vi "sub_GetNextState.vi"(4 "Stop":bool, 5 "Elapsed Time (sec)":dbl format="%#.2g", 6 "Start":bool, 7 "Car Position Slider":T1 scale=0.0..4.0, 8 "error in":errorcluster caption="에러 입력", 10 "Wash Options":T2, 11 "CurrentState":T3) -> (0 "error out":errorcluster caption="에러 출력", 3 "NextState":T3)   [LabVIEW 2018]
uses:
  Control/WashState.ctl
  Control/Wash Options.ctl
  Control/Car Position Control.ctl
  Control/Time.ctl
panel:
  out "결과":bool
  # "0"
  # "1"
  # "2"
  # "3"
  # "4"
  # "5"
  # "6"
  # "7"
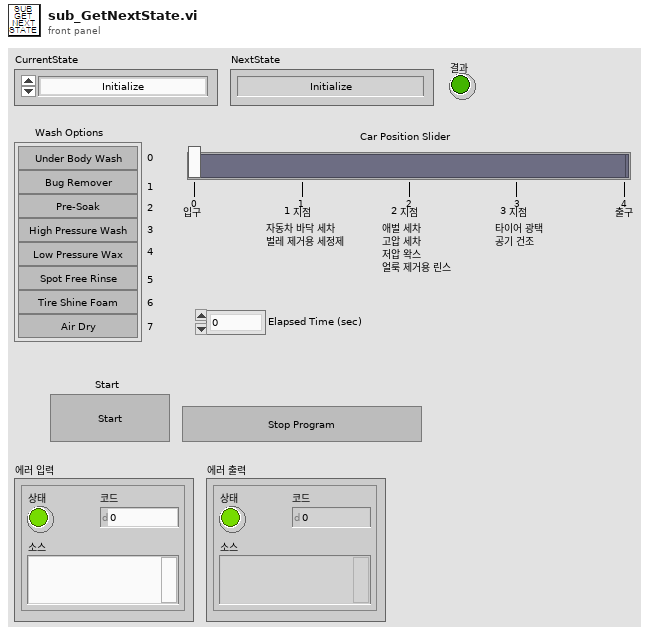
[diagram p1: front panel]
types:
  T1 = typedef "Car Position Control.ctl" = i32
  T2 = typedef "Wash Options.ctl" = cluster{"Under Body Wash":bool, "Bug Remover":bool, "Pre-Soak":bool, "High Pressure Wash":bool, "Low Pressure Wax":bool, "Spot Free Rinse":bool, "Tire Shine Foam":bool, "Air Dry":bool}
  T3 = typedef "WashState.ctl" = enum16{"Initialize", "Ready", "Under Body Wash", "Bug Remover", "Pre-Soak", "High Pressure Wash", "Low Pressure Wax", "Spot Free Rinse", "Tire Shine Foam", "Air Dry", "Stop", "Exit"}
  T4 = typedef "Time.ctl" = enum16{"Start", "End"}
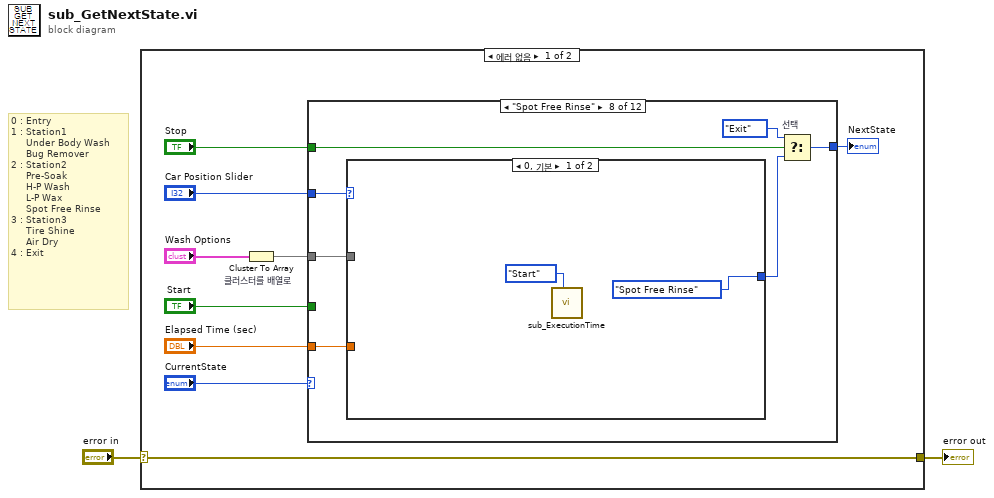
[diagram p0: block diagram]
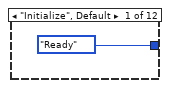
[diagram p2: hidden frame]
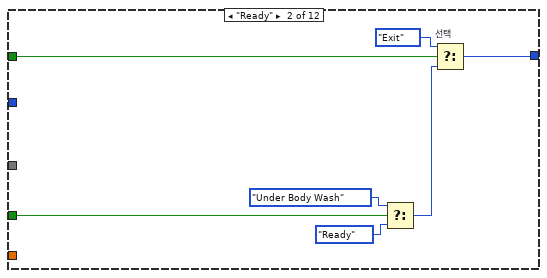
[diagram p3: hidden frame]
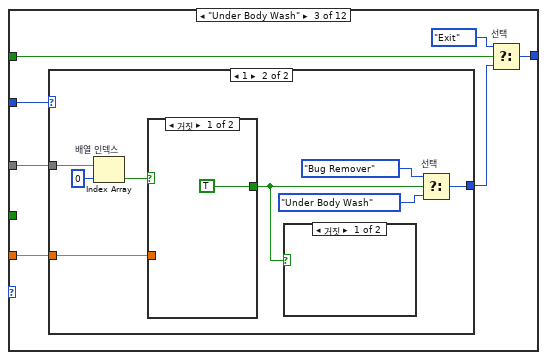
[diagram p4: hidden frame]
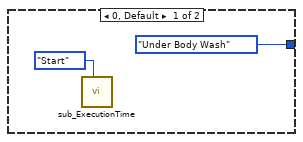
[diagram p5: hidden frame]
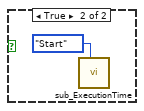
[diagram p6: hidden frame]
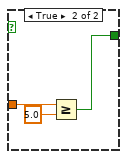
[diagram p7: hidden frame]
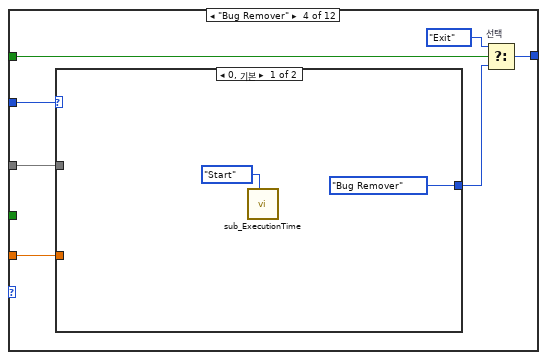
[diagram p8: hidden frame]
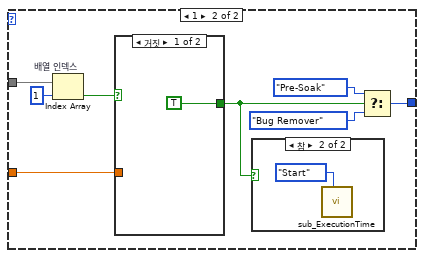
[diagram p9: hidden frame]
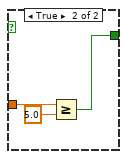
[diagram p11: hidden frame]
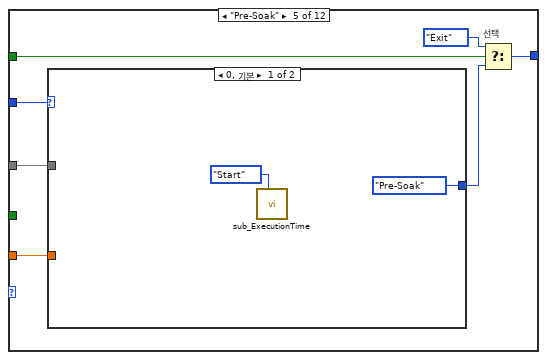
[diagram p12: hidden frame]
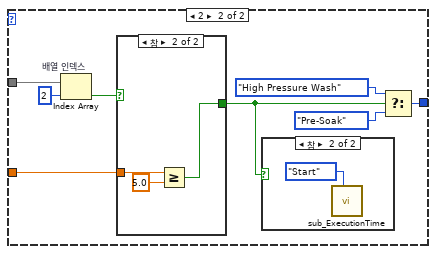
[diagram p13: hidden frame]
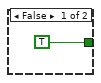
[diagram p15: hidden frame]
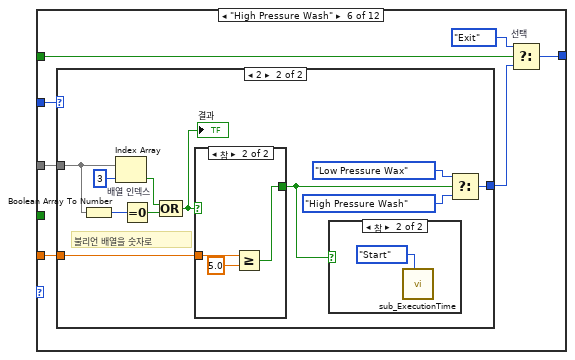
[diagram p16: hidden frame]
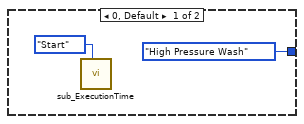
[diagram p17: hidden frame]
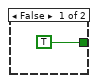
[diagram p19: hidden frame]
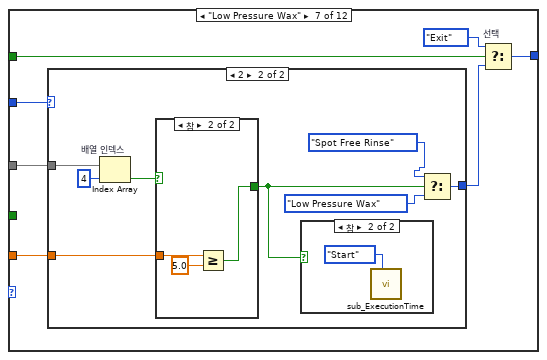
[diagram p20: hidden frame]
diagram:
  # "0 : Entry\n1 : Station1\n     Under Body Wash\n     Bug Remover\n2 : Station2\n     Pre-Soak\n     H-P Wash\n     L-P Wax\n     Spot Free Rinse\n3 : Station3\n     Tire Shine\n     Air Dry\n4 : Exit"
  n1 = case shown="에러 없음" "error in" {
    selector: "error in" -> [w11 w207]
    tunnel: [w11 w207] -> w1
    frame No Error {
      n2 = Cluster To Array "클러스터를 배열로"(cluster="Wash Options") -> (array=w7:bool[])
      n3 = case shown="\"Spot Free Rinse\"" "CurrentState" {
        tunnel: [WashState."Ready" ("NextState") w18 w25 w47 w69 w91 w116 w138 w160 w182 w202 WashState."Exit" ("NextState")] -> w9
        tunnel: w7 -> [_ _ w23 w45 w67 w89 w114 w136 w158 w180 _ _]
        tunnel: "Start" -> [_ w13 _ _ _ _ _ _ _ _ _ _]
        tunnel: "Stop" -> [_ w19 w26 w48 w70 w92 w117 w139 w161 w183 w203 _]
        tunnel: "Car Position Slider" -> [_ _ w21 w43 w65 w87 w112 w134 w156 w178 w199 _]
        tunnel: "Elapsed Time (sec)" -> [_ _ w20 w42 w64 w86 w111 w133 w155 w177 _ _]
        frame "Initialize", Default {
        }
        frame "Ready" {
          n4 = Select(t=WashState."Under Body Wash" ("NextState"), s=w13, f=WashState."Ready" ("NextState")) -> (s? t:f=w15:T3)
          n5 = Select "선택"(t=WashState."Exit" ("NextState"), s=w19, f=w15) -> (s? t:f=w18:T3)
        }
        frame "Under Body Wash" {
          n6 = case shown="1" w21 {
            tunnel: w23 -> [_ w36]
            tunnel: [WashState."Under Body Wash" ("NextState") w31] -> w22
            tunnel: w20 -> [_ w30]
            frame 0, Default {
              n7 = call "sub_ExecutionTime.vi"("State"=Time."Start") -> ()  [unwired: 9 in, 2 out]
            }
            frame 1 {
              n8 = Index Array "배열 인덱스"(array=w36, index=0 ("인덱스")) -> (element=w34:bool)
              n9 = case shown="거짓" w34 {
                tunnel: [TRUE ("Finish?") w39] -> w29
                tunnel: w30 -> [_ w41]
                frame False {
                }
                frame True {
                  n10 = Greater Or Equal?(x=w41, y=5.0) -> (x >= y?=w39:bool)
                }
              }
              n11 = case shown="거짓" w29 {
                frame False {
                }
                frame True {
                  n12 = call "sub_ExecutionTime.vi"("State"=Time."Start") -> ()  [unwired: 9 in, 2 out]
                }
              }
              n13 = Select "선택"(t=WashState."Bug Remover" ("NextState"), s=w29, f=WashState."Under Body Wash" ("NextState")) -> (s? t:f=w31:T3)
            }
          }
          n14 = Select "선택"(t=WashState."Exit" ("NextState"), s=w26, f=w22) -> (s? t:f=w25:T3)
        }
        frame "Bug Remover" {
          n15 = case shown="0, 기본" w43 {
            tunnel: w45 -> [_ w58]
            tunnel: [WashState."Bug Remover" ("NextState") w52] -> w44
            tunnel: w42 -> [_ w56]
            frame 0, Default {
              n16 = call "sub_ExecutionTime.vi"("State"=Time."Start") -> ()  [unwired: 9 in, 2 out]
            }
            frame 1 {
              n17 = Index Array "배열 인덱스"(array=w58, index=1 ("인덱스")) -> (element=w55:bool)
              n18 = case shown="거짓" w55 {
                tunnel: [TRUE ("Finish?") w61] -> w51
                tunnel: w56 -> [_ w63]
                frame False {
                }
                frame True {
                  n19 = Greater Or Equal?(x=w63, y=5.0) -> (x >= y?=w61:bool)
                }
              }
              n20 = case shown="참" w51 {
                frame False {
                }
                frame True {
                  n21 = call "sub_ExecutionTime.vi"("State"=Time."Start") -> ()  [unwired: 9 in, 2 out]
                }
              }
              n22 = Select(t=WashState."Pre-Soak" ("NextState"), s=w51, f=WashState."Bug Remover" ("NextState")) -> (s? t:f=w52:T3)
            }
          }
          n23 = Select "선택"(t=WashState."Exit" ("NextState"), s=w48, f=w44) -> (s? t:f=w47:T3)
        }
        frame "Pre-Soak" {
          n24 = case shown="0, 기본" w65 {
            tunnel: w67 -> [_ w80]
            tunnel: [WashState."Pre-Soak" ("NextState") w74] -> w66
            tunnel: w64 -> [_ w77]
            frame 0, Default {
              n25 = call "sub_ExecutionTime.vi"("State"=Time."Start") -> ()  [unwired: 9 in, 2 out]
            }
            frame 2 {
              n26 = Index Array "배열 인덱스"(array=w80, index=2 ("인덱스")) -> (element=w78:bool)
              n27 = case shown="참" w78 {
                tunnel: [TRUE ("Finish?") w83] -> w73
                tunnel: w77 -> [_ w85]
                frame False {
                }
                frame True {
                  n28 = Greater Or Equal?(x=w85, y=5.0) -> (x >= y?=w83:bool)
                }
              }
              n29 = case shown="참" w73 {
                frame False {
                }
                frame True {
                  n30 = call "sub_ExecutionTime.vi"("State"=Time."Start") -> ()  [unwired: 9 in, 2 out]
                }
              }
              n31 = Select(t=WashState."High Pressure Wash" ("NextState"), s=w73, f=WashState."Pre-Soak" ("NextState")) -> (s? t:f=w74:T3)
            }
          }
          n32 = Select "선택"(t=WashState."Exit" ("NextState"), s=w70, f=w66) -> (s? t:f=w69:T3)
        }
        frame "High Pressure Wash" {
          n33 = case shown="2" w87 {
            tunnel: w89 -> [_ w99]
            tunnel: [WashState."High Pressure Wash" ("NextState") w101] -> w88
            tunnel: w86 -> [_ w104]
            frame 0, Default {
              n34 = call "sub_ExecutionTime.vi"("State"=Time."Start") -> ()  [unwired: 9 in, 2 out]
            }
            frame 2 {
              # "불리언 배열을 숫자로"
              n35 = Boolean Array To Number(Boolean array=w99) -> (number=w98:u32)
              n36 = Index Array "배열 인덱스"(array=w99, index=3 ("인덱스")) -> (element=w97:bool)
              n37 = Equal To 0?(x=w98) -> (x = 0?=w96:bool)
              n38 = Compound Arithmetic op=OR(w97, w96) -> (w95:bool)
              "결과" <- w95
              n39 = case shown="참" w95 {
                tunnel: [TRUE ("Finish?") w108] -> w100
                tunnel: w104 -> [_ w110]
                frame False {
                }
                frame True {
                  n40 = Greater Or Equal?(x=w110, y=5.0) -> (x >= y?=w108:bool)
                }
              }
              n41 = case shown="참" w100 {
                frame False {
                }
                frame True {
                  n42 = call "sub_ExecutionTime.vi"("State"=Time."Start") -> ()  [unwired: 9 in, 2 out]
                }
              }
              n43 = Select(t=WashState."Low Pressure Wax" ("NextState"), s=w100, f=WashState."High Pressure Wash" ("NextState")) -> (s? t:f=w101:T3)
            }
          }
          n44 = Select "선택"(t=WashState."Exit" ("NextState"), s=w92, f=w88) -> (s? t:f=w91:T3)
        }
        frame "Low Pressure Wax" {
          n45 = case shown="2" w112 {
            tunnel: w114 -> [_ w127]
            tunnel: [WashState."Low Pressure Wax" ("NextState") w122] -> w113
            tunnel: w111 -> [_ w124]
            frame 0, Default {
              n46 = call "sub_ExecutionTime.vi"("State"=Time."Start") -> ()  [unwired: 9 in, 2 out]
            }
            frame 2 {
              n47 = Index Array "배열 인덱스"(array=w127, index=4 ("인덱스")) -> (element=w125:bool)
              n48 = case shown="참" w125 {
                tunnel: [TRUE ("Finish?") w130] -> w121
                tunnel: w124 -> [_ w132]
                frame False {
                }
                frame True {
                  n49 = Greater Or Equal?(x=w132, y=5.0) -> (x >= y?=w130:bool)
                }
              }
              n50 = case shown="참" w121 {
                frame False {
                }
                frame True {
                  n51 = call "sub_ExecutionTime.vi"("State"=Time."Start") -> ()  [unwired: 9 in, 2 out]
                }
              }
              n52 = Select(t=WashState."Spot Free Rinse" ("NextState"), s=w121, f=WashState."Low Pressure Wax" ("NextState")) -> (s? t:f=w122:T3)
            }
          }
          n53 = Select "선택"(t=WashState."Exit" ("NextState"), s=w117, f=w113) -> (s? t:f=w116:T3)
        }
        frame "Spot Free Rinse" {
          n54 = case shown="0, 기본" w134 {
            tunnel: w136 -> [_ w149]
            tunnel: [WashState."Spot Free Rinse" ("NextState") w144] -> w135
            tunnel: w133 -> [_ w146]
            frame 0, Default {
              n55 = call "sub_ExecutionTime.vi"("State"=Time."Start") -> ()  [unwired: 9 in, 2 out]
            }
            frame 2 {
              n56 = Index Array "배열 인덱스"(array=w149, index=5 ("인덱스")) -> (element=w147:bool)
              n57 = case shown="참" w147 {
                tunnel: [TRUE ("Finish?") w152] -> w143
                tunnel: w146 -> [_ w154]
                frame False {
                }
                frame True {
                  n58 = Greater Or Equal?(x=w154, y=5.0) -> (x >= y?=w152:bool)
                }
              }
              n59 = case shown="참" w143 {
                frame False {
                }
                frame True {
                  n60 = call "sub_ExecutionTime.vi"("State"=Time."Start") -> ()  [unwired: 9 in, 2 out]
                }
              }
              n61 = Select(t=WashState."Tire Shine Foam" ("NextState"), s=w143, f=WashState."Spot Free Rinse" ("NextState")) -> (s? t:f=w144:T3)
            }
          }
          n62 = Select "선택"(t=WashState."Exit" ("NextState"), s=w139, f=w135) -> (s? t:f=w138:T3)
        }
        frame "Tire Shine Foam" {
          n63 = case shown="0, 기본" w156 {
            tunnel: w158 -> [_ w171]
            tunnel: [WashState."Tire Shine Foam" ("NextState") w165] -> w157
            tunnel: w155 -> [_ w168]
            frame 0, Default {
              n64 = call "sub_ExecutionTime.vi"("State"=Time."Start") -> ()  [unwired: 9 in, 2 out]
            }
            frame 3 {
              n65 = Index Array "배열 인덱스"(array=w171, index=6 ("인덱스")) -> (element=w169:bool)
              n66 = case shown="참" w169 {
                tunnel: [TRUE ("Finish?") w174] -> w164
                tunnel: w168 -> [_ w176]
                frame False {
                }
                frame True {
                  n67 = Greater Or Equal?(x=w176, y=5.0) -> (x >= y?=w174:bool)
                }
              }
              n68 = case shown="참" w164 {
                frame False {
                }
                frame True {
                  n69 = call "sub_ExecutionTime.vi"("State"=Time."Start") -> ()  [unwired: 9 in, 2 out]
                }
              }
              n70 = Select(t=WashState."Air Dry" ("NextState"), s=w164, f=WashState."Tire Shine Foam" ("NextState")) -> (s? t:f=w165:T3)
            }
          }
          n71 = Select "선택"(t=WashState."Exit" ("NextState"), s=w161, f=w157) -> (s? t:f=w160:T3)
        }
        frame "Air Dry" {
          n72 = case shown="0, 기본" w178 {
            tunnel: w180 -> [_ w193]
            tunnel: [WashState."Air Dry" ("NextState") w187] -> w179
            tunnel: w177 -> [_ w190]
            frame 0, Default {
              n73 = call "sub_ExecutionTime.vi"("State"=Time."Start") -> ()  [unwired: 9 in, 2 out]
            }
            frame 3 {
              n74 = Index Array "배열 인덱스"(array=w193, index=7 ("인덱스")) -> (element=w191:bool)
              n75 = case shown="참" w191 {
                tunnel: [TRUE ("Finish?") w196] -> w186
                tunnel: w190 -> [_ w198]
                frame False {
                }
                frame True {
                  n76 = Greater Or Equal?(x=w198, y=5.0) -> (x >= y?=w196:bool)
                }
              }
              n77 = case shown="참" w186 {
                frame False {
                }
                frame True {
                  n78 = call "sub_ExecutionTime.vi"("State"=Time."Start") -> ()  [unwired: 9 in, 2 out]
                }
              }
              n79 = Select(t=WashState."Stop" ("NextState"), s=w186, f=WashState."Air Dry" ("NextState")) -> (s? t:f=w187:T3)
            }
          }
          n80 = Select "선택"(t=WashState."Exit" ("NextState"), s=w183, f=w179) -> (s? t:f=w182:T3)
        }
        frame "Stop" {
          n81 = case shown="4" w199 {
            tunnel: [WashState."Stop" ("NextState") WashState."Ready" ("NextState")] -> w200
            frame 0, Default {
            }
            frame 4 {
            }
          }
          n82 = Select "선택"(t=WashState."Exit" ("NextState"), s=w203, f=w200) -> (s? t:f=w202:T3)
        }
        frame "Exit" {
        }
      }
      "NextState" <- w9
    }
    frame Error {
    }
  }
  "error out" <- w1
